vi "MS SQL_Routing.vi"(11 "data":variant[][](array[variant])) -> (3 "Array":bool[](array[boolean]))   [LabVIEW 2020]
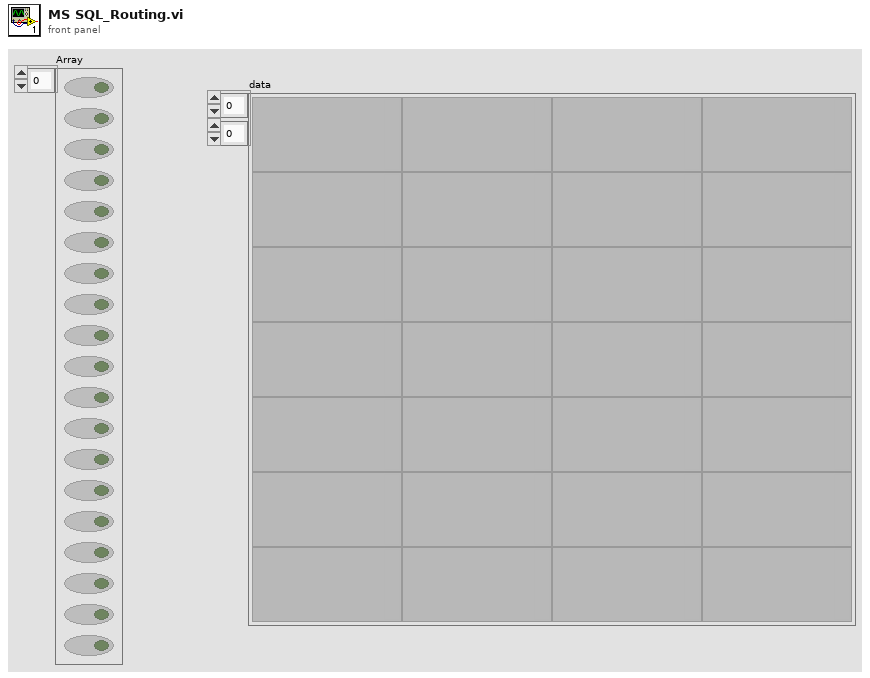
[diagram p1: front panel]
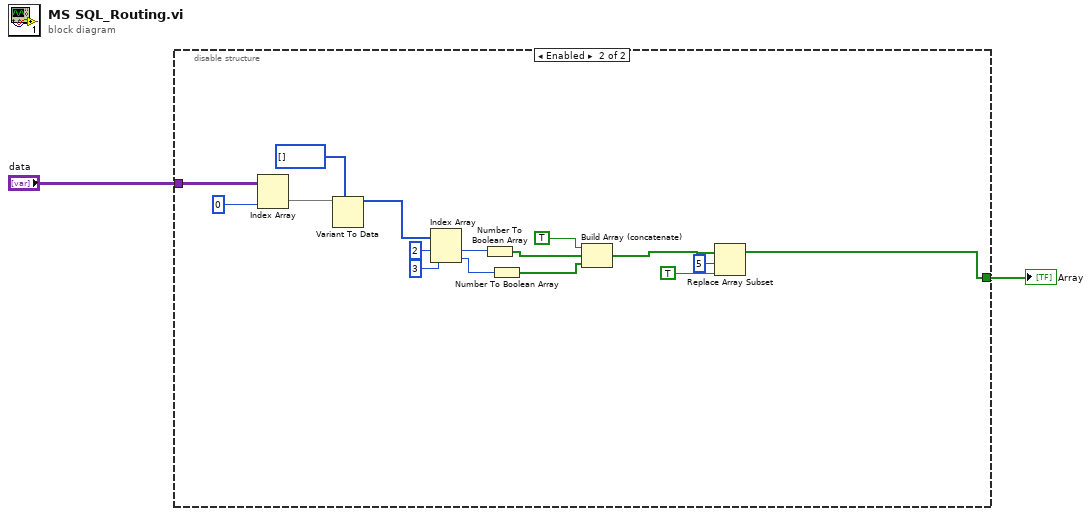
[diagram p0: block diagram]
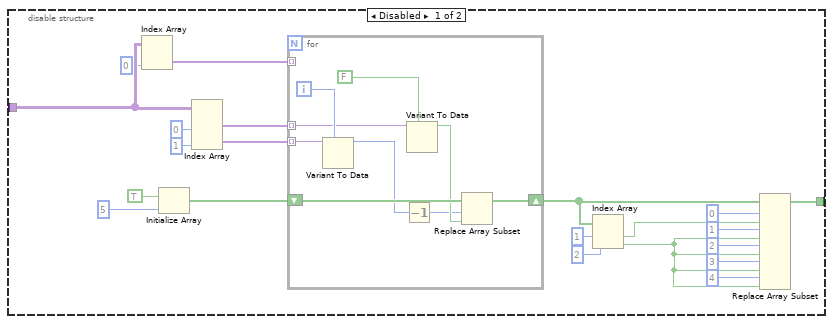
[diagram p2: hidden frame]
diagram:
  n1 = disable-structure shown="Enabled" {
    disable-tunnel: "data" -> [w16 w48]
    disable-tunnel: [w11 w35] -> w1
    frame Disabled {
      n2 = Index Array(array=w16, index (col)=0 ("disabled index (col)")) -> (element=w15:variant[])  [unwired: 1 in]
      n3 = Initialize Array(TRUE, 5 ("dimension size")) -> (w23:bool[])
      n4 = Index Array(array=w16, index (col) #1=0 ("disabled index (col)"), index (col) #2=1 ("index (col)")) -> (element #1=w18:variant[], element #2=w20:variant[])  [unwired: 2 in]
      n5 = for {
        tunnel: w18 -> [w26] mode=indexing
        tunnel: w20 -> [w32] mode=indexing
        shift-right: [w24] -> w12
        shift-left: w23 -> [w30]
        tunnel: w15 -> [_] mode=indexing
        i -> [w31]
        n6 = Variant To Data(type=w31, Variant=w32) -> (data=w28:i32)  [unwired: 1 in, 1 out]
        n7 = Decrement(x=w28) -> (x-1=w25:i32)
        n8 = Variant To Data(type=FALSE, Variant=w26) -> (data=w29:bool)  [unwired: 1 in, 1 out]
        n9 = Replace Array Subset(array=w30, new element=w29, index=w25) -> (w24:bool[])
      }
      n10 = Index Array(array=w12, index #1=1 ("index"), index #2=2 ("index")) -> (element #1=w9:bool, element #2=w3:bool)
      n11 = Replace Array Subset(array=w12, new element #1=w9, index #1=0 ("index"), new element #2=w3, index #2=1 ("index"), new element #3=w3, index #3=2 ("index"), new element #4=w3, index #4=3 ("index"), new element #5=w3, index #5=4 ("index")) -> (w11:bool[])
    }
    frame Enabled {
      n12 = Index Array(array=w48, index (col)=0 ("disabled index (col)")) -> (element=w46:variant[])  [unwired: 1 in]
      n13 = Variant To Data(type=i32[] [], Variant=w46) -> (data=w44:i32[])  [unwired: 1 in, 1 out]
      n14 = Index Array(array=w44, index #1=2 ("index"), index #2=3 ("index")) -> (element #1=w42:i32, element #2=w38:i32)
      n15 = Number To Boolean Array(number=w42) -> (Boolean array=w41:bool[])
      n16 = Number To Boolean Array(number=w38) -> (Boolean array=w37:bool[])
      n17 = Build Array (concatenate)(TRUE, w41, w37) -> (w36:bool[])
      n18 = Replace Array Subset(array=w36, new element=TRUE ("new element/subarray"), index=5) -> (w35:bool[])
    }
  }
  "Array" <- w1
